vi "FPGA.vi"() -> ()   [LabVIEW 2015]
uses:
  <vilib>/rvi/Emulation/niFpgaGetClockAttributes.vi
  <vilib>/rvi/Emulation/niFpgaSctlEmulationGetInTimedLoop.vi
  <vilib>/rvi/Emulation/niFpgaEmulationReportErrorSimple.vi
  <vilib>/rvi/eio/common/nirviEmuTemplateMethod_errors.vi
  <vilib>/rvi/DataTransferAndStorage/Container/Common/niFpgaContainerGetUniqueNameForEmu.vi
  <vilib>/rvi/DataTransferAndStorage/Container/Common/niFpgaContainerSetEmuInfo.vi
  <vilib>/rvi/eio/common/nirviEmuReportErrorAndStop.vi
  <vilib>/rvi/DataTransferAndStorage/Container/Common/niFpgaContainerExecOnDevCompGetState.vi
  <vilib>/rvi/Emulation/niFpgaEmulationIsFPGAContextNoSignature.vi
  <vilib>/rvi/errors/niFpgaSetErrorForExecOnDevCompSimple.vi
  <vilib>/rvi/FIFO/Fifo_Resource/nirvififoEmulationSetSize.vi
  <vilib>/rvi/FIFO/Fifo_Resource/nirviFifoEmulationQueueMgr.vi
  <instcachedir>/0/nirviFifoEmulationQueueMgr_E5CAEC123FF24DC58D834DCA3CDAA9B5.lvgen/nirviFifoEmulationQueueMgr_E5CAEC123FF24DC58D834DCA3CDAA9B5_001.vi
  <vilib>/rvi/FIFO/Fifo_Resource/nirvififoEmulationDetermineInputValidOut.vi
  <vilib>/rvi/FIFO/Fifo_Resource/nirvififoEmulationCreateLock.vi
  <vilib>/rvi/Emulation/niFpgaProcessEmulError.vi
  <vilib>/rvi/FIFO/Fifo_Resource/nirvififoEmulationObtainLock.vi
  <vilib>/rvi/FIFO/Fifo_Resource/nirvififoEmulationReleaseLock.vi
  <vilib>/rvi/occurrence/nirviWaitOnOccurrenceBase.vi
  <vilib>/rvi/errors/nirviReportUnexpectedCaseInternalError.vi
  <vilib>/rvi/errors/nirviReportUnexpectedCaseInternalError (U32).vi
  <vilib>/Utility/error.llb/Clear Errors.vi
  <vilib>/rvi/interface/RandomDataEmulation/niFpgaRandomDataHandleErrors.vi
  <instcachedir>/0/nirviFifoEmulationQueueMgr_E5CAEC123FF24DC58D834DCA3CDAA9B5.lvgen/nirviFifoEmulationQueueMgr_E5CAEC123FF24DC58D834DCA3CDAA9B5_002.vi
  <vilib>/rvi/Emulation/niFpgaCriticalErrorInLSC.vi
  <vilib>/eio/EIONode/EIONode.xnode
  <vilib>/rvi/LocalResourceManager/LocalResourceManager.xnode
  <vilib>/rvi/DataTransferAndStorage/Container/XNode/niFpgaContainer.xnode
  <vilib>/rvi/FIFO/Fifo_Resource/niFpgaFifoEmulationRefIn.vi
panel:
  out "a8":u16
  out "a7":u16
  out "a6":u16
  out "d2":bool
  out "d1":bool
  out "d3":bool
  out "a5":u16
  out "a4":u16
  out "a3":u16
  out "a2":u16
  out "State":T1(ring)
  out "a1":u16
  out "pased":bool
  in  "pedir":bool
  out "ready":bool
  in  "pasar":bool
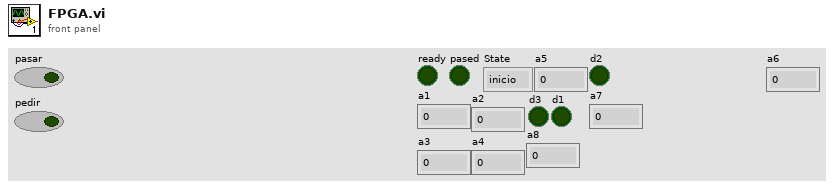
[diagram p1: front panel]
types:
  T1 = enum16{"inicio", "muestreo", "finMuestreo", "peticion", "envio"}
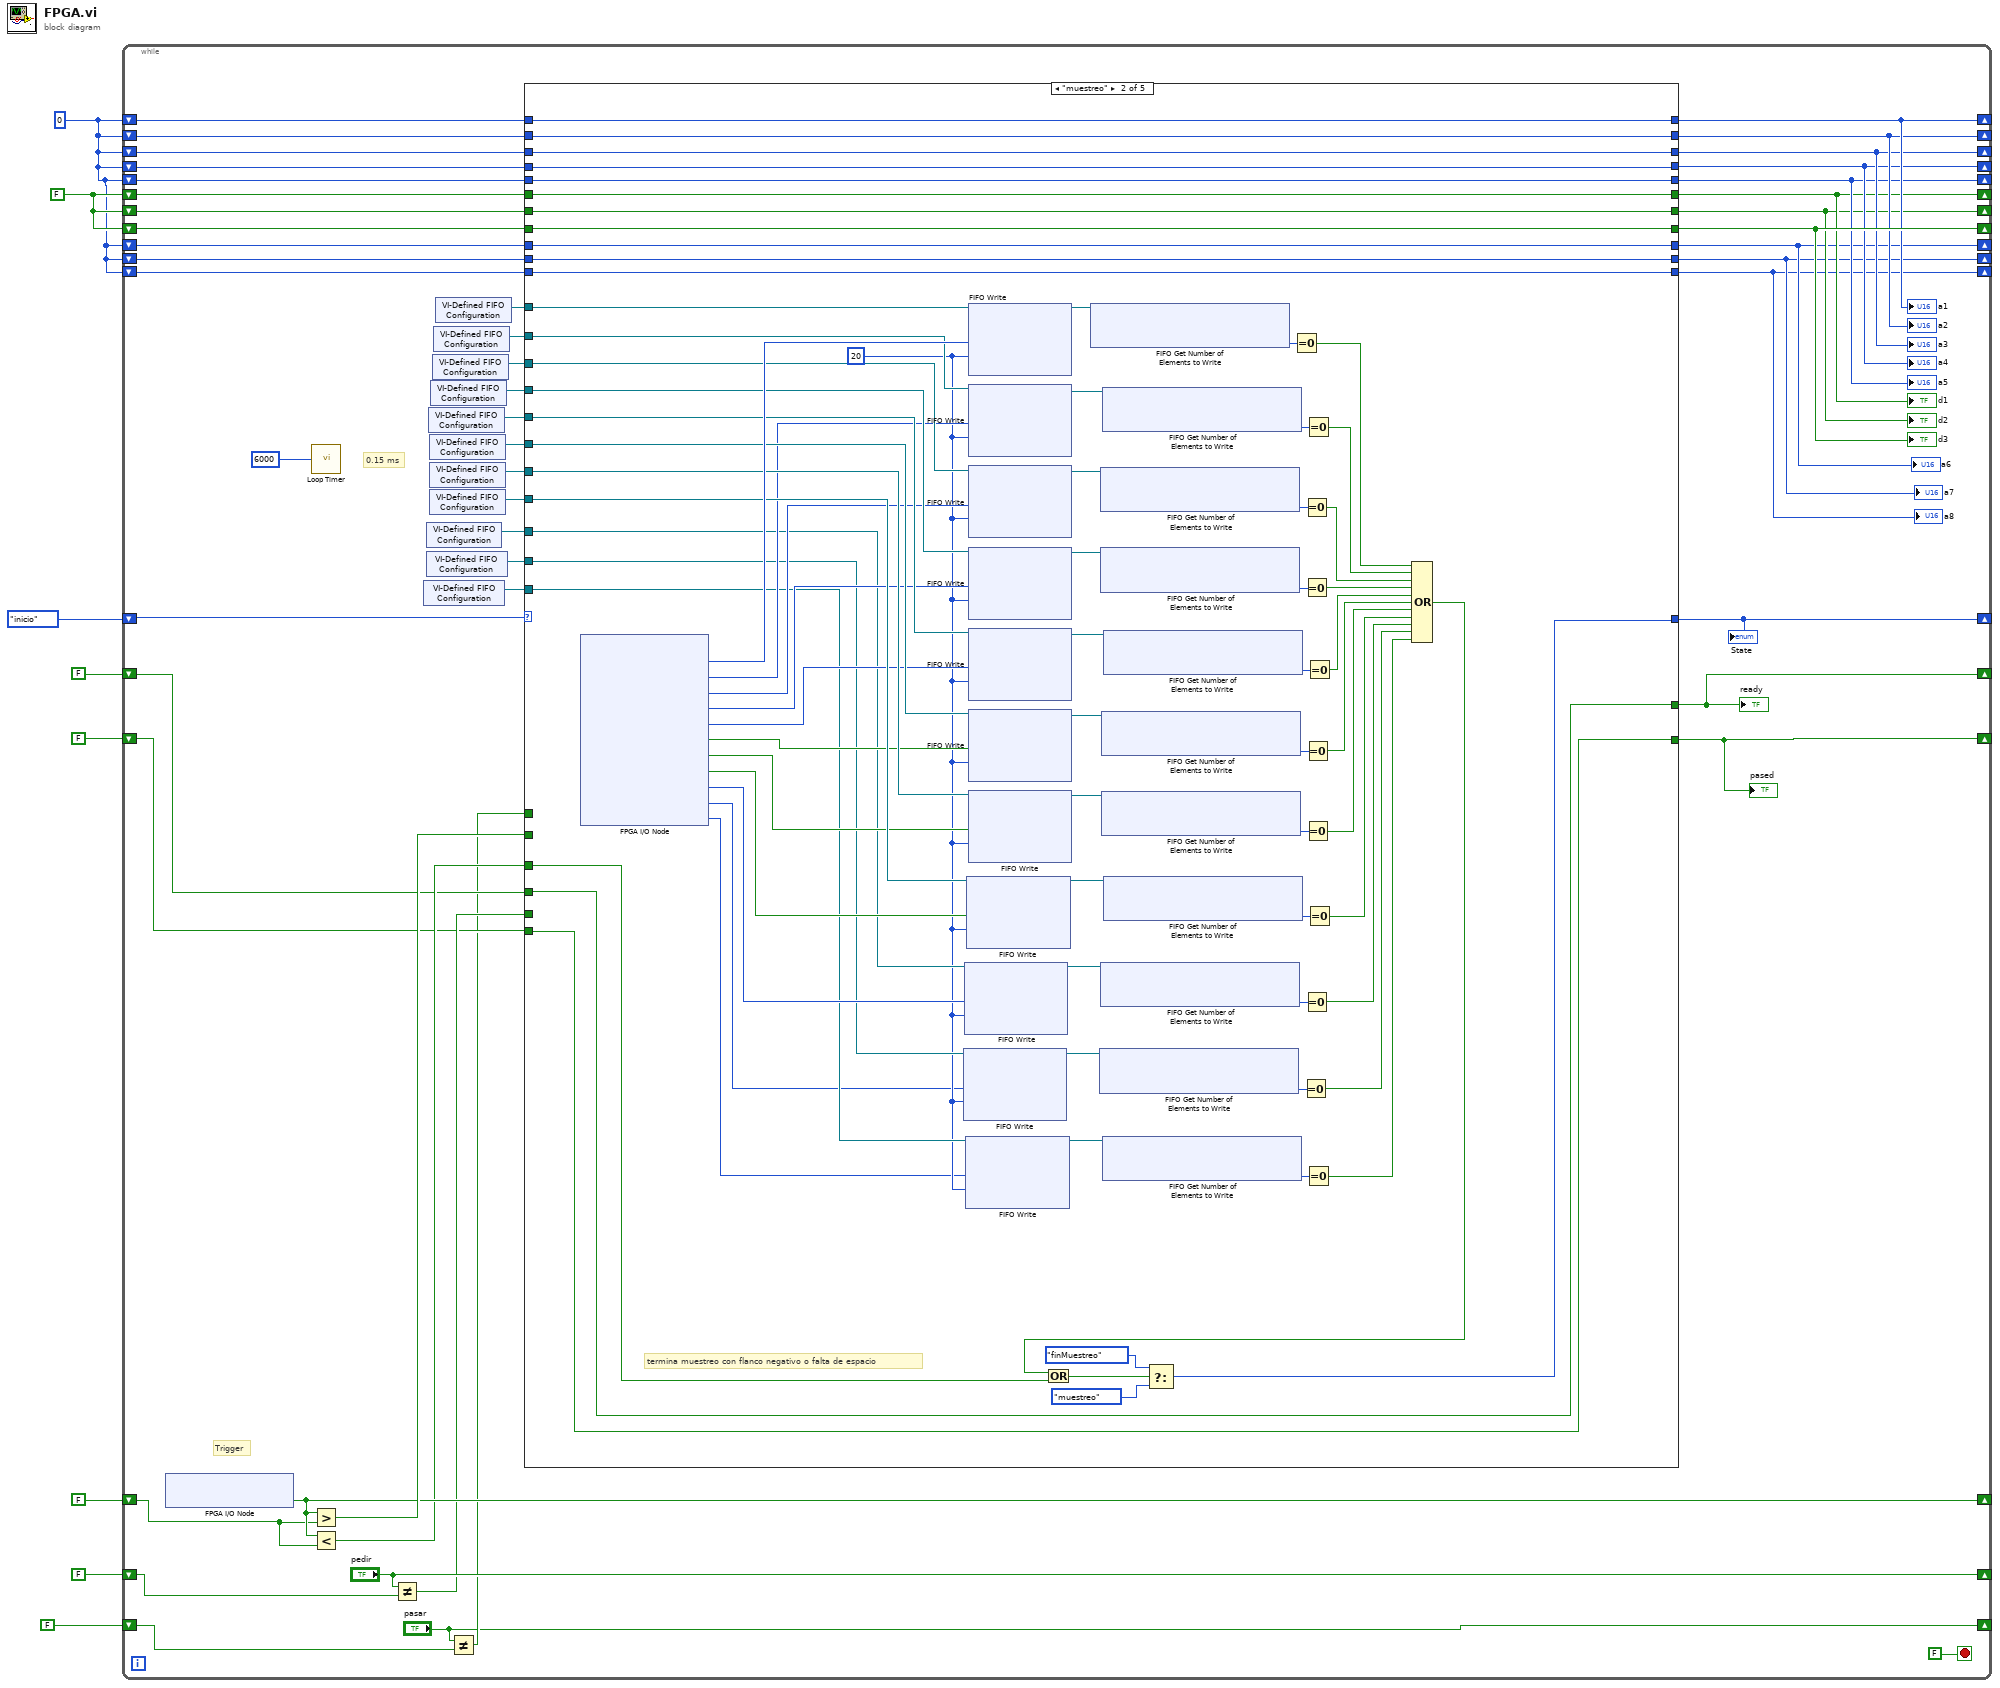
[diagram p0: block diagram]
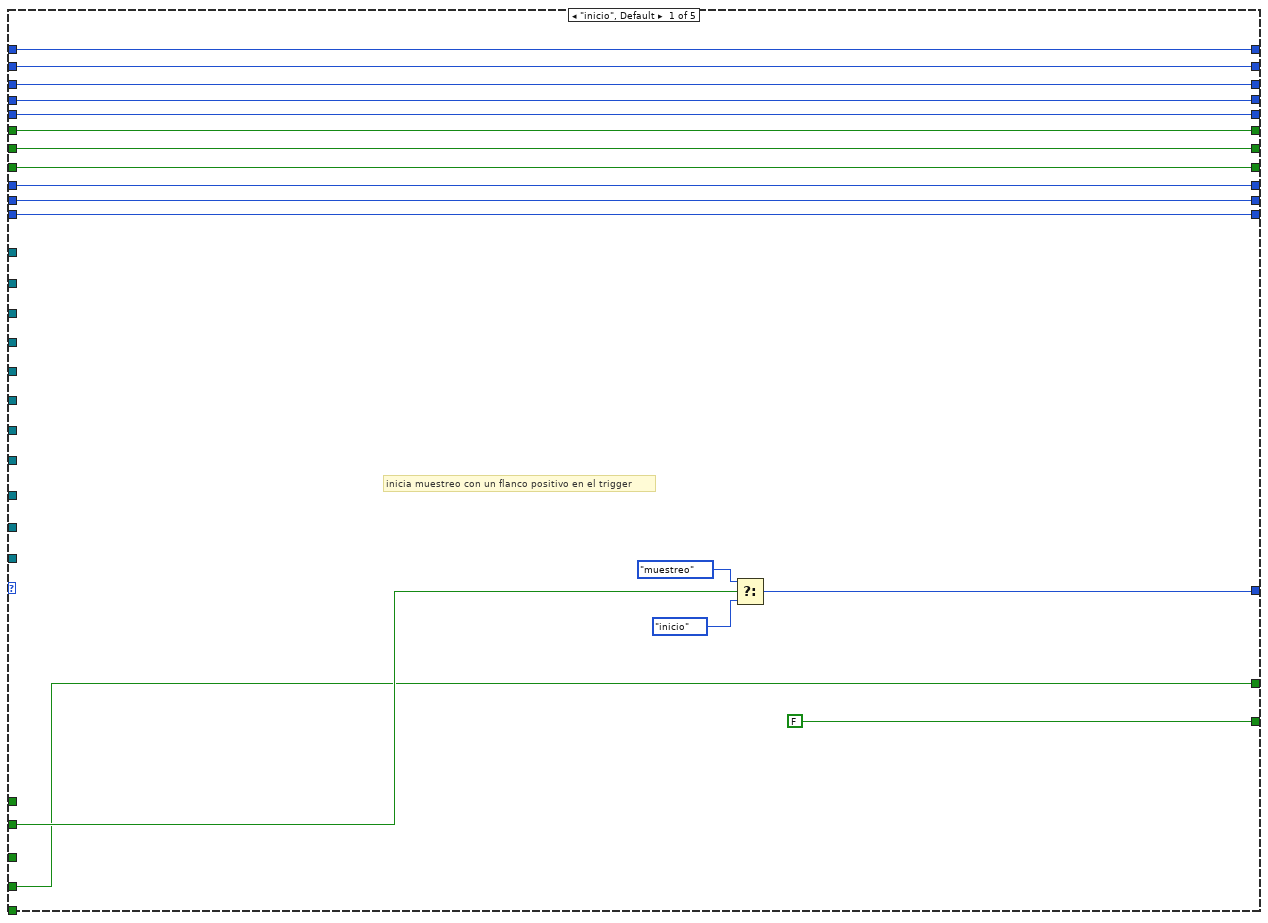
[diagram p2: hidden frame]
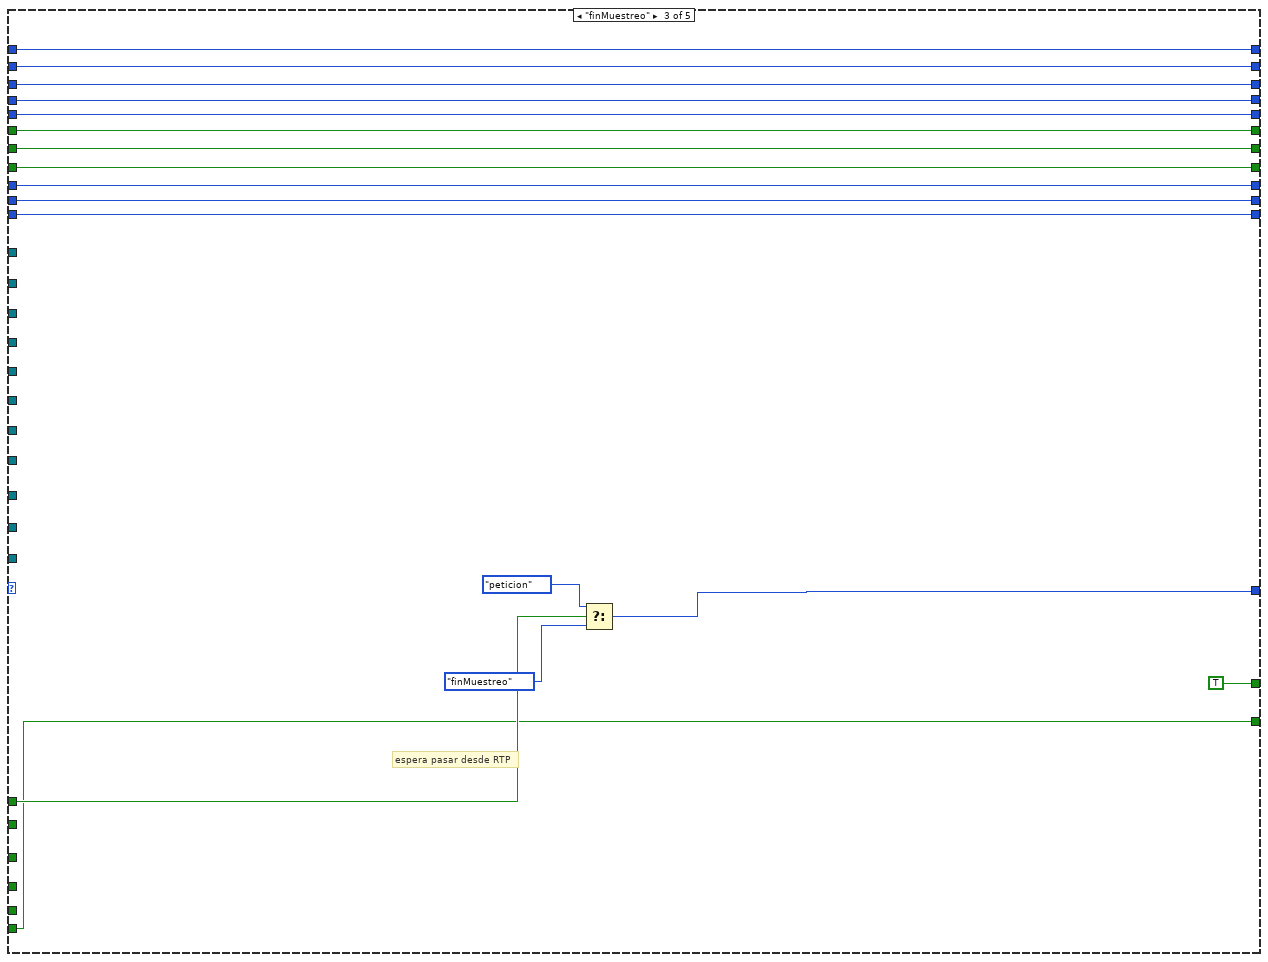
[diagram p3: hidden frame]
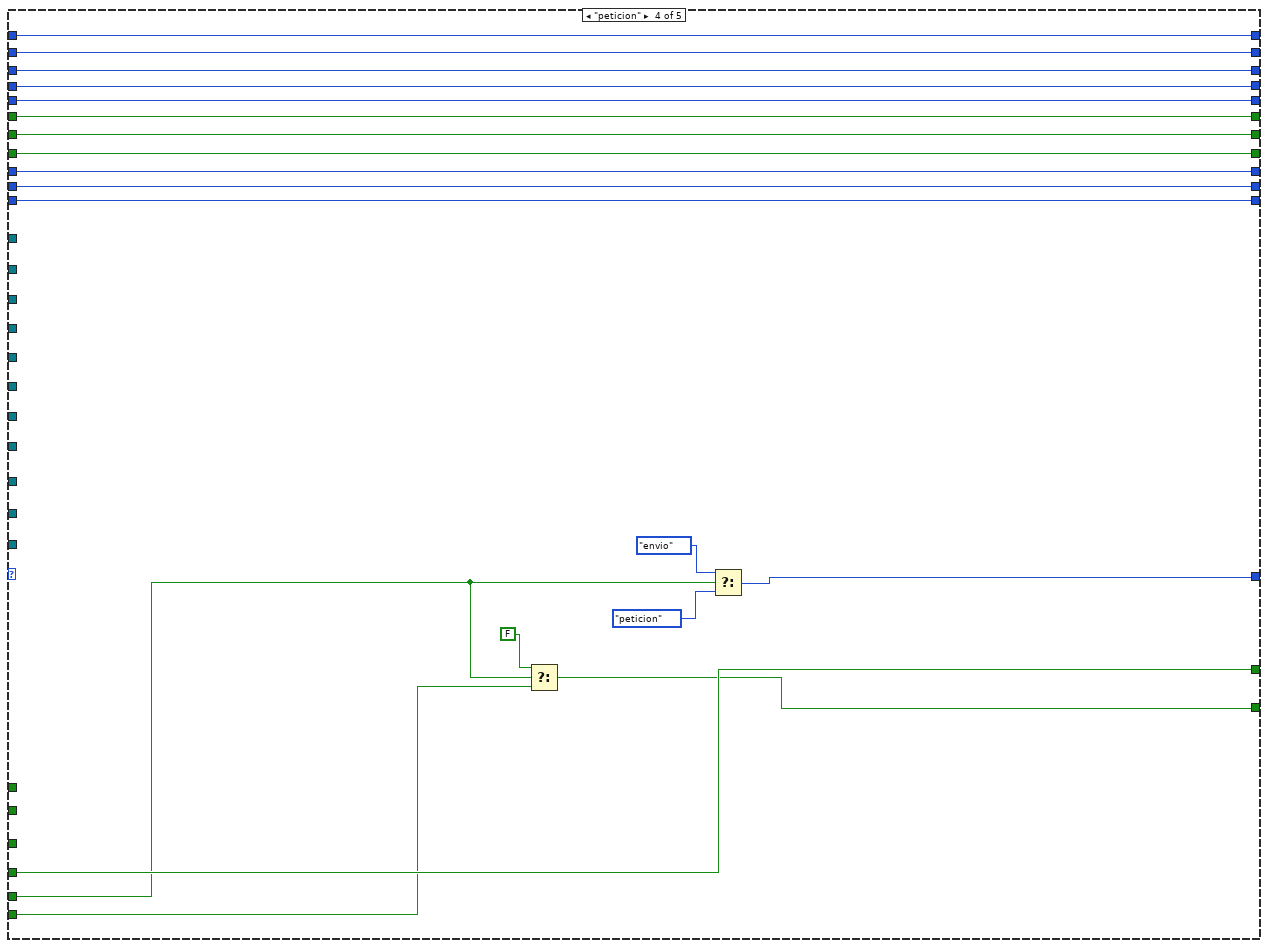
[diagram p4: hidden frame]
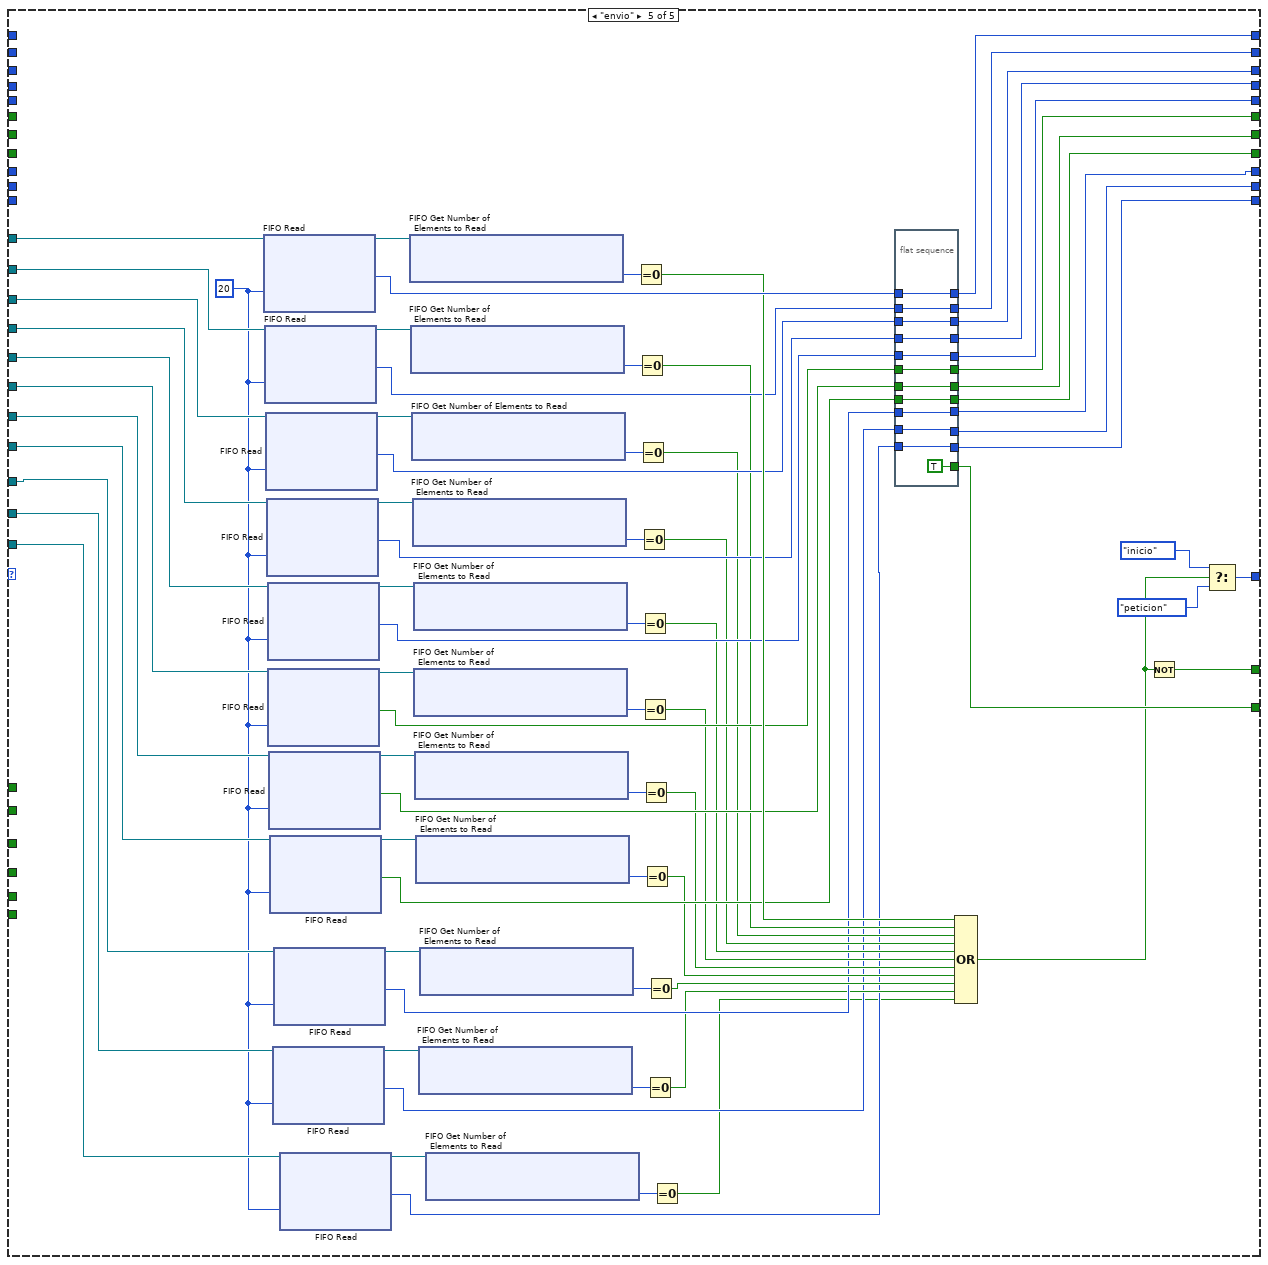
[diagram p5: hidden frame]
diagram:
  w2 = FALSE ("Element")
  w1 = u16 0 ("Element")
  n1 = while {
    shift-right: [w54] -> _
    shift-left: FALSE ("ConnectorA/DIO0") -> [w53]
    shift-right: [w57] -> _
    shift-left: T1."inicio" -> [w58]
    shift-right: ["pedir"] -> _
    shift-left: FALSE ("pedir") -> [w50]
    shift-right: [w48] -> _
    shift-left: FALSE -> [w47]
    shift-right: [w46] -> _
    shift-left: FALSE -> [w45]
    shift-right: ["pasar"] -> _
    shift-left: FALSE ("pasar") -> [w43]
    shift-right: [w24] -> _
    shift-left: w1 -> [w32]
    shift-right: [w23] -> _
    shift-left: w1 -> [w31]
    shift-right: [w22] -> _
    shift-left: w1 -> [w30]
    shift-right: [w21] -> _
    shift-left: w1 -> [w29]
    shift-right: [w20] -> _
    shift-left: w1 -> [w28]
    shift-right: [w19] -> _
    shift-left: w2 -> [w27]
    shift-right: [w18] -> _
    shift-left: w2 -> [w26]
    shift-right: [w33] -> _
    shift-left: w2 -> [w25]
    shift-right: [w15] -> _
    shift-left: w1 -> [w16]
    shift-right: [w10] -> _
    shift-left: w1 -> [w12]
    shift-right: [w9] -> _
    shift-left: w1 -> [w11]
    stop <- FALSE stop-if-true
    # "0.15 ms"
    # "Trigger"
    n2 = xnode "FPGA I/O Node"() -> ("ConnectorA/DIO3"=w54:bool)  [unwired: 1 in, 1 out]
    n3 = call "Loop Timer"("Count(Ticks)"=u32 6000) -> ()  [unwired: 1 out]
    n4 = Greater?(x=w54, y=w53) -> (0:w56:bool)
    n5 = Less?(x=w54, y=w53) -> (x < y?=w52:bool)
    n6 = Not Equal?(x="pedir", y=w50) -> (x != y?=w49:bool)
    n7 = xnode "VI-Defined FIFO Configuration"() -> ("FIFO Out"=w13:refnum<k21>)
    n8 = xnode "VI-Defined FIFO Configuration"() -> ("FIFO Out"=w17:refnum<k21>)
    n9 = xnode "VI-Defined FIFO Configuration"() -> ("FIFO Out"=w14:refnum<k21>)
    n10 = xnode "VI-Defined FIFO Configuration"() -> ("FIFO Out"=w39:refnum<k21>)
    n11 = xnode "VI-Defined FIFO Configuration"() -> ("FIFO Out"=w38:refnum<k21>)
    n12 = xnode "VI-Defined FIFO Configuration"() -> ("FIFO Out"=w37:refnum<k21>)
    n13 = xnode "VI-Defined FIFO Configuration"() -> ("FIFO Out"=w36:refnum<k21>)
    n14 = xnode "VI-Defined FIFO Configuration"() -> ("FIFO Out"=w40:refnum<k21>)
    n15 = xnode "VI-Defined FIFO Configuration"() -> ("FIFO Out"=w41:refnum<k21>)
    n16 = xnode "VI-Defined FIFO Configuration"() -> ("FIFO Out"=w42:refnum<k21>)
    n17 = xnode "VI-Defined FIFO Configuration"() -> ("FIFO Out"=w55:refnum<k21>)
    n18 = Not Equal?(x="pasar", y=w43) -> (x != y?=w35:bool)
    n19 = case shown="\"muestreo\"" w58 {
      tunnel: [w73 w143 w165 w185 w258] -> w57
      tunnel: w56 -> [w74 _ _ _ _]
      tunnel: w55 -> [_ w151 _ _ w255]
      tunnel: w52 -> [_ w146 _ _ _]
      tunnel: w35 -> [_ _ w168 _ _]
      tunnel: [w72 w142 TRUE w184 w230] -> w48
      tunnel: w49 -> [_ _ _ w183 _]
      tunnel: [FALSE w104 w163 w181 w256] -> w46
      tunnel: w47 -> [w72 w142 _ w184 _]
      tunnel: w45 -> [_ w104 w163 w180 _]
      tunnel: w42 -> [_ w141 _ _ w249]
      tunnel: w41 -> [_ w140 _ _ w246]
      tunnel: w40 -> [_ w139 _ _ w245]
      tunnel: w39 -> [_ w138 _ _ w240]
      tunnel: w38 -> [_ w137 _ _ w237]
      tunnel: w37 -> [_ w136 _ _ w234]
      tunnel: w36 -> [_ w135 _ _ w231]
      tunnel: [w70 w103 w162 w179 w214] -> w24
      tunnel: [w69 w102 w161 w178 w213] -> w23
      tunnel: [w68 w101 w160 w177 w212] -> w22
      tunnel: [w67 w100 w159 w176 w211] -> w21
      tunnel: [w66 w99 w158 w175 w210] -> w20
      tunnel: [w65 w98 w157 w174 w209] -> w19
      tunnel: [w64 w97 w156 w173 w208] -> w18
      tunnel: [w63 w96 w155 w172 w207] -> w33
      tunnel: w32 -> [w70 w103 w162 w179 _]
      tunnel: w31 -> [w69 w102 w161 w178 _]
      tunnel: w30 -> [w68 w101 w160 w177 _]
      tunnel: w29 -> [w67 w100 w159 w176 _]
      tunnel: w28 -> [w66 w99 w158 w175 _]
      tunnel: w27 -> [w65 w98 w157 w174 _]
      tunnel: w26 -> [w64 w97 w156 w173 _]
      tunnel: w25 -> [w63 w96 w155 w172 _]
      tunnel: w17 -> [_ w92 _ _ w204]
      tunnel: w16 -> [w62 w79 w154 w171 _]
      tunnel: [w62 w79 w154 w171 w201] -> w15
      tunnel: w14 -> [_ w86 _ _ w196]
      tunnel: w13 -> [_ w85 _ _ w194]
      tunnel: [w61 w78 w153 w170 w189] -> w10
      tunnel: [w60 w77 w152 w169 w188] -> w9
      tunnel: w12 -> [w61 w78 w153 w170 _]
      tunnel: w11 -> [w60 w77 w152 w169 _]
      frame "inicio", Default {
        # "inicia muestreo con un flanco positivo en el trigger"
        n20 = Select(t=T1."muestreo", s=w74, f=T1."inicio") -> (s? t:f=w73:T1)
      }
      frame "muestreo" {
        w84 = 20 ("Timeout")
        # "termina muestreo con flanco negativo o falta de espacio"
        n21 = xnode "FPGA I/O Node"() -> ("ConnectorA/AI0"=w150:u16, "ConnectorA/AI1"=w111:u16, "ConnectorA/AI2"=w110:u16, "ConnectorA/AI3"=w109:u16, "ConnectorB/AI0"=w108:u16, "ConnectorA/DIO0"=w107:bool, "ConnectorA/DIO1"=w106:bool, "ConnectorA/DIO2"=w105:bool, "ConnectorB/AI1"=w91:u16, "ConnectorB/AI2"=w83:u16, "ConnectorB/AI3"=w82:u16)  [unwired: 11 in, 11 out]
        n22 = xnode ("FIFO Write")("Element"=w83, "Timeout"=w84, "FIFO In"=w86) -> ("FIFO Out"=w89:refnum<k21>)  [unwired: 1 out]
        n23 = xnode ("FIFO Write")("Element"=w91, "Timeout"=w84, "FIFO In"=w92) -> ("FIFO Out"=w95:refnum<k21>)  [unwired: 1 out]
        n24 = xnode ("FIFO Write")("Element"=w82, "Timeout"=w84, "FIFO In"=w85) -> ("FIFO Out"=w88:refnum<k21>)  [unwired: 1 out]
        n25 = xnode ("FIFO Write")("Element"=w105, "Timeout"=w84, "FIFO In"=w135) -> ("FIFO Out"=w121:refnum<k21>)  [unwired: 1 out]
        n26 = xnode ("FIFO Write")("Element"=w150, "Timeout"=w84, "FIFO In"=w151) -> ("FIFO Out"=w149:refnum<k21>)  [unwired: 1 out]
        n27 = xnode ("FIFO Write")("Element"=w111, "Timeout"=w84, "FIFO In"=w141) -> ("FIFO Out"=w126:refnum<k21>)  [unwired: 1 out]
        n28 = xnode ("FIFO Write")("Element"=w110, "Timeout"=w84, "FIFO In"=w140) -> ("FIFO Out"=w127:refnum<k21>)  [unwired: 1 out]
        n29 = xnode ("FIFO Write")("Element"=w109, "Timeout"=w84, "FIFO In"=w139) -> ("FIFO Out"=w125:refnum<k21>)  [unwired: 1 out]
        n30 = xnode ("FIFO Write")("Element"=w108, "Timeout"=w84, "FIFO In"=w138) -> ("FIFO Out"=w124:refnum<k21>)  [unwired: 1 out]
        n31 = xnode ("FIFO Write")("Element"=w107, "Timeout"=w84, "FIFO In"=w137) -> ("FIFO Out"=w123:refnum<k21>)  [unwired: 1 out]
        n32 = xnode ("FIFO Write")("Element"=w106, "Timeout"=w84, "FIFO In"=w136) -> ("FIFO Out"=w122:refnum<k21>)  [unwired: 1 out]
        n33 = xnode ("FIFO Get Number of Elements to Write")("FIFO In"=w149) -> ("Number of Elements to Write"=w148:u32)  [unwired: 1 out]
        n34 = xnode ("FIFO Get Number of Elements to Write")("FIFO In"=w89) -> ("Number of Elements to Write"=w90:u32)  [unwired: 1 out]
        n35 = xnode ("FIFO Get Number of Elements to Write")("FIFO In"=w127) -> ("Number of Elements to Write"=w133:u32)  [unwired: 1 out]
        n36 = xnode ("FIFO Get Number of Elements to Write")("FIFO In"=w125) -> ("Number of Elements to Write"=w132:u32)  [unwired: 1 out]
        n37 = xnode ("FIFO Get Number of Elements to Write")("FIFO In"=w95) -> ("Number of Elements to Write"=w94:u32)  [unwired: 1 out]
        n38 = xnode ("FIFO Get Number of Elements to Write")("FIFO In"=w123) -> ("Number of Elements to Write"=w130:u32)  [unwired: 1 out]
        n39 = xnode ("FIFO Get Number of Elements to Write")("FIFO In"=w122) -> ("Number of Elements to Write"=w129:u32)  [unwired: 1 out]
        n40 = xnode ("FIFO Get Number of Elements to Write")("FIFO In"=w126) -> ("Number of Elements to Write"=w134:u32)  [unwired: 1 out]
        n41 = xnode ("FIFO Get Number of Elements to Write")("FIFO In"=w88) -> ("Number of Elements to Write"=w87:u32)  [unwired: 1 out]
        n42 = xnode ("FIFO Get Number of Elements to Write")("FIFO In"=w124) -> ("Number of Elements to Write"=w131:u32)  [unwired: 1 out]
        n43 = xnode ("FIFO Get Number of Elements to Write")("FIFO In"=w121) -> ("Number of Elements to Write"=w128:u32)  [unwired: 1 out]
        n44 = Equal To 0?(x=w148) -> (x = 0?=w120:bool)
        n45 = Equal To 0?(x=w90) -> (x = 0?=w81:bool)
        n46 = Equal To 0?(x=w133) -> (x = 0?=w118:bool)
        n47 = Equal To 0?(x=w132) -> (x = 0?=w117:bool)
        n48 = Equal To 0?(x=w94) -> (x = 0?=w93:bool)
        n49 = Equal To 0?(x=w130) -> (x = 0?=w115:bool)
        n50 = Equal To 0?(x=w129) -> (x = 0?=w114:bool)
        n51 = Equal To 0?(x=w134) -> (x = 0?=w119:bool)
        n52 = Equal To 0?(x=w87) -> (x = 0?=w80:bool)
        n53 = Equal To 0?(x=w131) -> (x = 0?=w116:bool)
        n54 = Equal To 0?(x=w128) -> (x = 0?=w113:bool)
        n55 = Compound Arithmetic op=OR(w120, w119, w118, w117, w116, w115, w114, w113, w93, w81, w80) -> (w112:bool)
        n56 = Or(x=w112, y=w146) -> (x .or. y?=w147:bool)
        n57 = Select(t=T1."finMuestreo", s=w147, f=T1."muestreo") -> (s? t:f=w143:T1)
      }
      frame "finMuestreo" {
        # "espera pasar desde RTP"
        n58 = Select(t=T1."peticion", s=w168, f=T1."finMuestreo") -> (s? t:f=w165:T1)
      }
      frame "peticion" {
        n59 = Select(t=FALSE, s=w183, f=w180) -> (s? t:f=w181:bool)
        n60 = Select(t=T1."envio", s=w183, f=T1."peticion") -> (s? t:f=w185:T1)
      }
      frame "envio" {
        w193 = 20 ("Timeout")
        n61 = xnode ("FIFO Read")("Timeout"=w193, "FIFO In"=w255) -> ("Element"=w253:u16, "FIFO Out"=w254:refnum<k21>)  [unwired: 1 out]
        n62 = xnode ("FIFO Read")("Timeout"=w193, "FIFO In"=w249) -> ("Element"=w229:u16, "FIFO Out"=w251:refnum<k21>)  [unwired: 1 out]
        n63 = xnode ("FIFO Read")("Timeout"=w193, "FIFO In"=w246) -> ("Element"=w228:u16, "FIFO Out"=w247:refnum<k21>)  [unwired: 1 out]
        n64 = xnode ("FIFO Read")("Timeout"=w193, "FIFO In"=w245) -> ("Element"=w227:u16, "FIFO Out"=w244:refnum<k21>)  [unwired: 1 out]
        n65 = xnode ("FIFO Read")("Timeout"=w193, "FIFO In"=w240) -> ("Element"=w226:u16, "FIFO Out"=w241:refnum<k21>)  [unwired: 1 out]
        n66 = xnode ("FIFO Read")("Timeout"=w193, "FIFO In"=w237) -> ("Element"=w225:bool, "FIFO Out"=w239:refnum<k21>)  [unwired: 1 out]
        n67 = xnode ("FIFO Read")("Timeout"=w193, "FIFO In"=w234) -> ("Element"=w224:bool, "FIFO Out"=w235:refnum<k21>)  [unwired: 1 out]
        n68 = xnode ("FIFO Read")("Timeout"=w193, "FIFO In"=w231) -> ("Element"=w223:bool, "FIFO Out"=w233:refnum<k21>)  [unwired: 1 out]
        n69 = xnode ("FIFO Read")("Timeout"=w193, "FIFO In"=w196) -> ("Element"=w192:u16, "FIFO Out"=w200:refnum<k21>)  [unwired: 1 out]
        n70 = xnode ("FIFO Read")("Timeout"=w193, "FIFO In"=w204) -> ("Element"=w202:u16, "FIFO Out"=w205:refnum<k21>)  [unwired: 1 out]
        n71 = xnode ("FIFO Read")("Timeout"=w193, "FIFO In"=w194) -> ("Element"=w191:u16, "FIFO Out"=w197:refnum<k21>)  [unwired: 1 out]
        n72 = xnode ("FIFO Get Number of Elements to Read")("FIFO In"=w254) -> ("Number of Elements to Read"=w257:u32)  [unwired: 1 out]
        n73 = xnode ("FIFO Get Number of Elements to Read")("FIFO In"=w251) -> ("Number of Elements to Read"=w250:u32)  [unwired: 1 out]
        n74 = xnode ("FIFO Get Number of Elements to Read")("FIFO In"=w247) -> ("Number of Elements to Read"=w248:u32)  [unwired: 1 out]
        n75 = xnode ("FIFO Get Number of Elements to Read")("FIFO In"=w244) -> ("Number of Elements to Read"=w243:u32)  [unwired: 1 out]
        n76 = xnode ("FIFO Get Number of Elements to Read")("FIFO In"=w241) -> ("Number of Elements to Read"=w242:u32)  [unwired: 1 out]
        n77 = xnode ("FIFO Get Number of Elements to Read")("FIFO In"=w239) -> ("Number of Elements to Read"=w238:u32)  [unwired: 1 out]
        n78 = xnode ("FIFO Get Number of Elements to Read")("FIFO In"=w235) -> ("Number of Elements to Read"=w236:u32)  [unwired: 1 out]
        n79 = xnode ("FIFO Get Number of Elements to Read")("FIFO In"=w233) -> ("Number of Elements to Read"=w232:u32)  [unwired: 1 out]
        n80 = xnode ("FIFO Get Number of Elements to Read")("FIFO In"=w200) -> ("Number of Elements to Read"=w199:u32)  [unwired: 1 out]
        n81 = xnode ("FIFO Get Number of Elements to Read")("FIFO In"=w205) -> ("Number of Elements to Read"=w206:u32)  [unwired: 1 out]
        n82 = xnode ("FIFO Get Number of Elements to Read")("FIFO In"=w197) -> ("Number of Elements to Read"=w198:u32)  [unwired: 1 out]
        n83 = Equal To 0?(x=w257) -> (x = 0?=w252:bool)
        n84 = Equal To 0?(x=w250) -> (x = 0?=w221:bool)
        n85 = Equal To 0?(x=w248) -> (x = 0?=w220:bool)
        n86 = Equal To 0?(x=w243) -> (x = 0?=w219:bool)
        n87 = Equal To 0?(x=w242) -> (x = 0?=w218:bool)
        n88 = Equal To 0?(x=w238) -> (x = 0?=w217:bool)
        n89 = Equal To 0?(x=w236) -> (x = 0?=w216:bool)
        n90 = Equal To 0?(x=w232) -> (x = 0?=w215:bool)
        n91 = Equal To 0?(x=w199) -> (x = 0?=w195:bool)
        n92 = Equal To 0?(x=w206) -> (x = 0?=w203:bool)
        n93 = Equal To 0?(x=w198) -> (x = 0?=w190:bool)
        n94 = flat-sequence {
          tunnel: [TRUE] -> w256
          tunnel: w253 -> [w271]
          tunnel: [w271] -> w214
          tunnel: [w270] -> w213
          tunnel: w229 -> [w270]
          tunnel: w228 -> [w269]
          tunnel: [w269] -> w212
          tunnel: [w268] -> w211
          tunnel: w227 -> [w268]
          tunnel: w226 -> [w267]
          tunnel: w225 -> [w264]
          tunnel: w224 -> [w266]
          tunnel: w223 -> [w265]
          tunnel: [w267] -> w210
          tunnel: [w266] -> w208
          tunnel: [w265] -> w207
          tunnel: [w264] -> w209
          tunnel: w202 -> [w263]
          tunnel: [w263] -> w201
          tunnel: w192 -> [w262]
          tunnel: w191 -> [w261]
          tunnel: [w262] -> w189
          tunnel: [w261] -> w188
          frame #0 {
          }
        }
        n95 = Compound Arithmetic op=OR(w252, w221, w220, w219, w218, w217, w216, w215, w203, w195, w190) -> (w222:bool)
        n96 = Not(x=w222) -> (.not. x?=w230:bool)
        n97 = Select(t=T1."inicio", s=w222, f=T1."peticion") -> (s? t:f=w258:T1)
      }
    }
    "ready" <- w48
    "pased" <- w46
    "a1" <- w24
    "State" <- w57
    "a2" <- w23
    "a3" <- w22
    "a4" <- w21
    "a5" <- w20
    "d3" <- w33
    "d1" <- w19
    "d2" <- w18
    "a6" <- w15
    "a7" <- w10
    "a8" <- w9
  }
